vi "Configure Instrument.vi"(0 "VISA resource name":refnum<visa-resource-name>, 5 "Remote Interface\nMode (0: Local)":u16(ring) items=["Local", "Remote", "Remote w/ Lockout"], 7 "Lock-Out (F: Off)":bool, 9 "Lock-Out Code (123)":dbl=123.0 min=0.0 max=999.0 step=1.0, 11 "error in (no error)":errorcluster, 12 "Beeper (F: Off)":bool) -> (4 "VISA resource name out":refnum<visa-resource-name>, 15 "error out":errorcluster)   [LabVIEW 2013, in "Lake Shore Cryotronics 331.lvlib"]
doc: "This VI configures various instrument settings. Parameters configured are;\nRemote interface mode, Keypad lock out, Audible beeper status."
uses:
  Lake Shore Cryotronics 331.lvlib
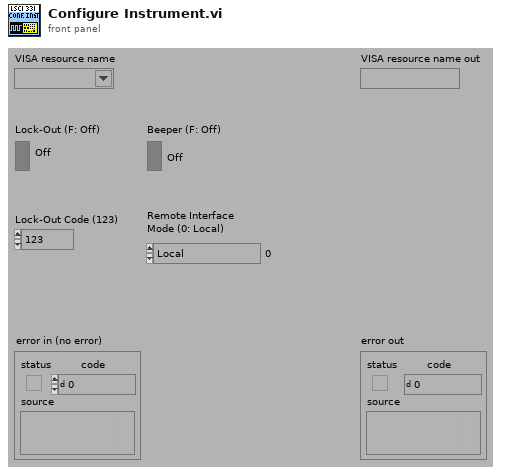
[diagram p1: front panel]
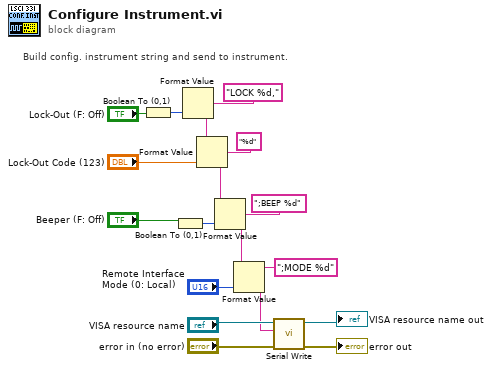
[diagram p0: block diagram]
diagram:
  # "Build config. instrument string and send to instrument."
  n1 = Boolean To (0,1)(Boolean="Lock-Out (F: Off)") -> (0, 1=w15:i16)
  n2 = Boolean To (0,1)(Boolean="Beeper (F: Off)") -> (0, 1=w11:i16)
  n3 = Format Value(format string="LOCK %d,", value (0)=w15) -> (output string=w12:string)  [unwired: 1 in]
  n4 = Format Value(string ("")=w12, format string="%d", value (0)="Lock-Out Code (123)") -> (output string=w3:string)
  n5 = Format Value(string ("")=w3, format string=";BEEP %d", value (0)=w11) -> (output string=w2:string)
  n6 = Format Value(string ("")=w2, format string=";MODE %d", value (0)="Remote Interface\nMode (0: Local)") -> (output string=w4:string)
  n7 = call "Serial Write.vi"("error in (no error)"="error in (no error)", "Write Buffer (\"\")"=w4, "VISA resource name"="VISA resource name") -> ("error out"=→"error out":errorcluster, "VISA resource name out"=→"VISA resource name out":refnum<visa-resource-name>)  [unwired: 6 in, 1 out]
